vi "getFPGA.vi"(11 "OuterLoopClockIRQ in":refnum<class "OuterLoopClockIRQ.lvclass">) -> (2 "FPGA":refnum<class "FPGA.lvclass">, 3 "OuterLoopClockIRQ out":refnum<class "OuterLoopClockIRQ.lvclass">)   [LabVIEW 2016, in "OuterLoopClockIRQ.lvclass"]
uses:
  OuterLoopClockIRQ.lvclass
  FPGA/FPGA.lvclass
  OuterLoopClockIRQ.lvclass/OuterLoopClockIRQ.ctl
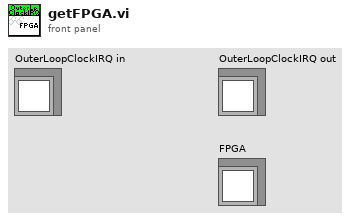
[diagram p1: front panel]
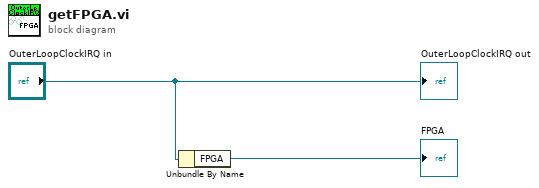
[diagram p0: block diagram]
diagram:
  n1 = Unbundle By Name("OuterLoopClockIRQ in") -> ("FPGA"=→"FPGA":refnum<class "FPGA.lvclass">)
  "OuterLoopClockIRQ out" <- "OuterLoopClockIRQ in"
